vi "NumIntegrate_Trap_Mat.vi"(8 "dT":dbl=0.02, 9 "Prev Y":T1, 10 "Y":T1, 11 "Prev_Integral":T1) -> (1 "New Prev Y":T1, 3 "Integral":T1)   [LabVIEW 2019, in "Trajectory_Library.lvlib"]
doc: "Performs the calculation for trapezoidal integration of matrices. The previous value of X is not stored inside this function The user is responsible for this.\n\nInputs:\n - Prev_Integral -- The current value of the integrated matrix\n - Y -- Current value of Y matrix\n - Prev Y -- The previous value of Y matrix.\n - dT -- Time interval over which to integrate\n\nOutputs:\n - Integral -- Updated integrated output matrix\n - New Prev Y -- The previous value of Y to use the next iteration matrix."
uses:
  Trajectory_Library.lvlib
  <vilib>/Analysis/Matrix/Datatypes/RealMatrix.ctl
  <vilib>/Analysis/Matrix/Numeric/Add/Add - RM,RM.vi
  <vilib>/Analysis/Matrix/Numeric/Multiply/Multiply - RM,R.vi
  <vilib>/Analysis/Matrix/NI_Matrix.lvlib
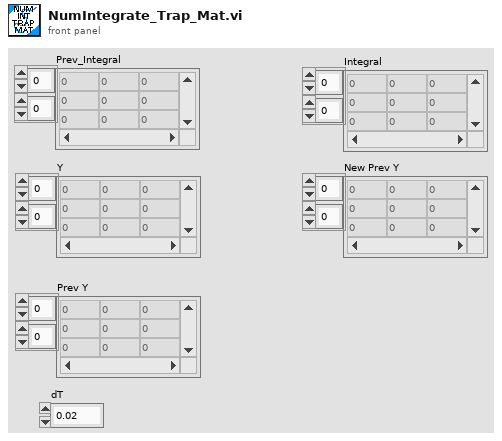
[diagram p1: front panel]
types:
  T1 = typedef "NI_Matrix.lvlib/RealMatrix.ctl" = dbl[][]
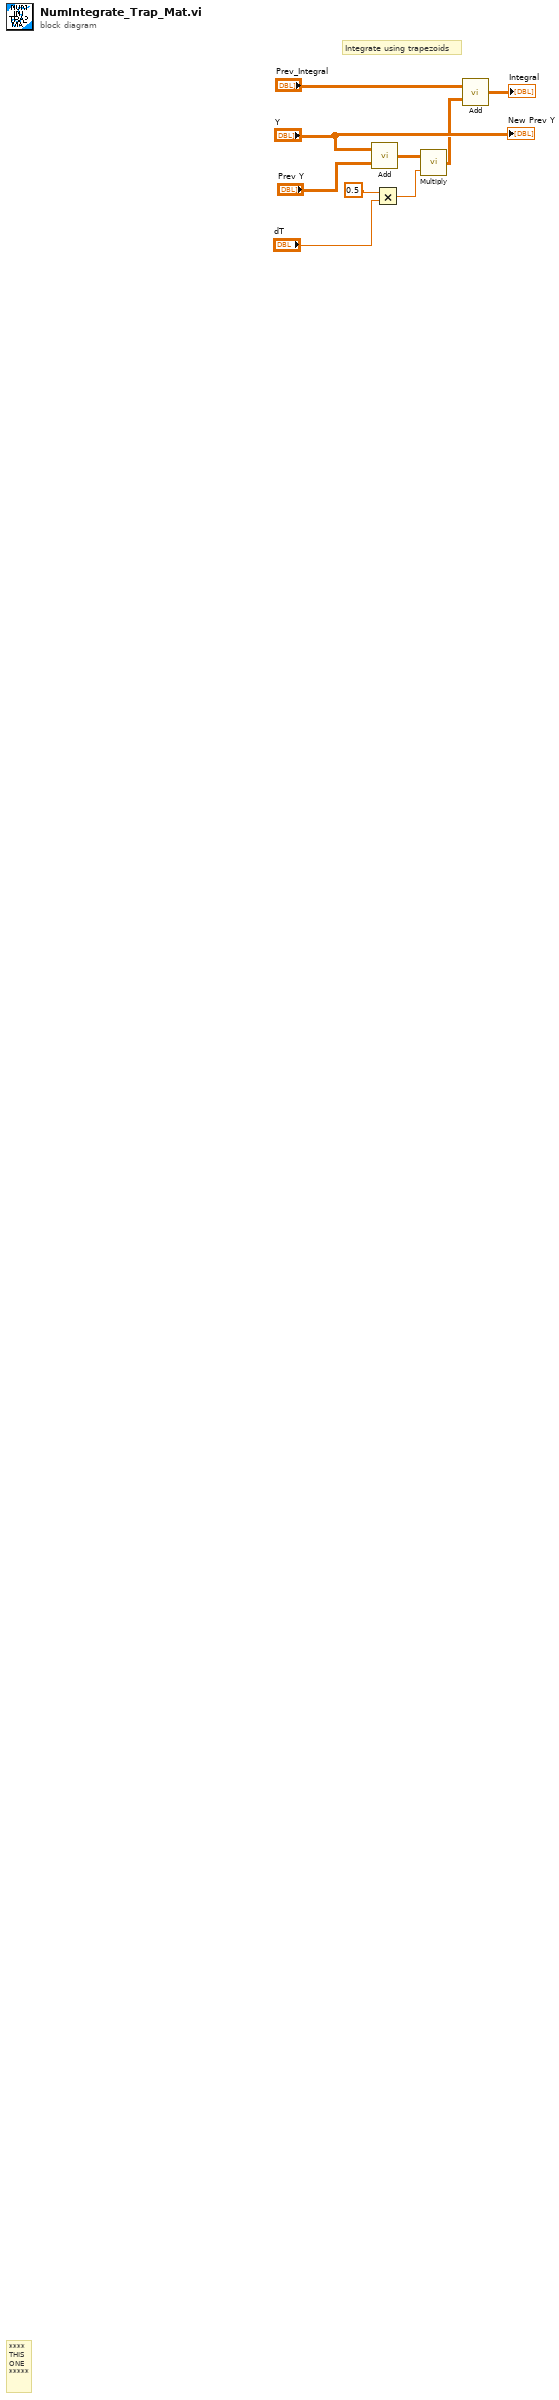
[diagram p0: block diagram]
diagram:
  # "Integrate using trapezoids"
  # "****\nTHIS\nONE\n*****"
  n1 = call-poly <vilib>:"Add.vi"("Real Matrix B"="Prev Y", "Real Matrix A"="Y") -> ("A + B"=w2:T1)
  n2 = Multiply(x=0.5 ("value"), y="dT") -> (x*y=w1:dbl)
  n3 = call-poly <vilib>:"Multiply.vi"("Real Scalar c"=w1, "Real Matrix A"=w2) -> ("A * c"=w7:T1)
  n4 = call-poly <vilib>:"Add.vi"("Real Matrix B"=w7, "Real Matrix A"="Prev_Integral") -> ("A + B"=→"Integral":T1)
  "New Prev Y" <- "Y"
